vi "Get Temp Control--Method.vi"(8 "Error In":errorcluster, 11 "Watlow F4T in":refnum<class "Watlow F4T.lvclass">) -> (0 "Error Out":errorcluster, 1 "Output":dbl, 2 "Control State":bool, 3 "Watlow F4T out":refnum<class "Watlow F4T.lvclass">)   [LabVIEW 2024, in "Watlow F4T.lvclass"]
uses:
  Watlow F4T.lvclass
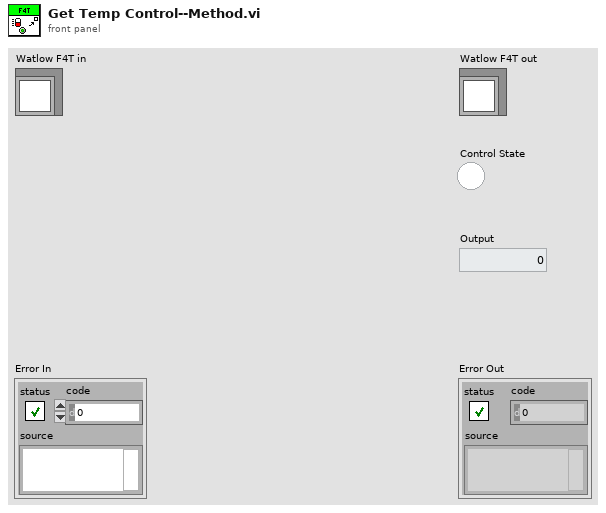
[diagram p1: front panel]
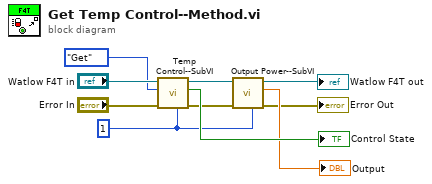
[diagram p0: block diagram]
diagram:
  w1 = 1 ("Instance")
  n1 = call "Temp Control--SubVI.vi"("Instance"=w1, "error in"="Error In", "Get/Set"=enum16{"Get", "Set"}."Get", "Watlow F4T in"="Watlow F4T in") -> ("error out"=w6:errorcluster, "Temp Control"=→"Control State":bool, "Watlow F4T out"=w5:refnum<class "Watlow F4T.lvclass">)  [unwired: 5 in]
  n2 = call "Output Power--SubVI.vi"("Instance(1)"=w1, "error in (no error)"=w6, "Watlow F4T In"=w5) -> ("error out"=→"Error Out":errorcluster, "Output (+/-100%)"=→"Output":dbl, "Watlow F4T out"=→"Watlow F4T out":refnum<class "Watlow F4T.lvclass">)  [unwired: 6 in]
